vi "twoWire_Resistance_test.vi"() -> ()   [LabVIEW 2026]
uses:
  <vilib>/regexp/Match Regular Expression.xnode
panel:
  out "R (Ohm)":dbl
  in  "VISA resource name":refnum<visa-resource-name>
  out "raw response":string
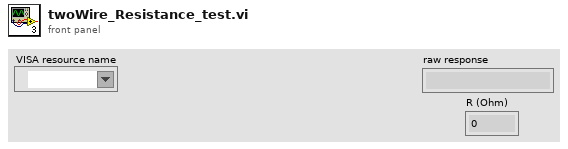
[diagram p1: front panel]
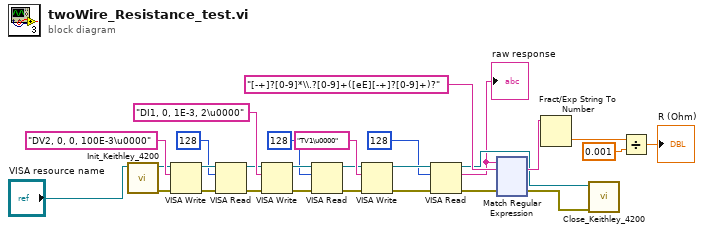
[diagram p0: block diagram]
diagram:
  n1 = call "Init_Keithley_4200.vi"("VISA resource name"="VISA resource name") -> ("error out"=w12:errorcluster, "VISA resource name out"=w13:refnum<visa-resource-name>)  [unwired: 9 in]
  n2 = VISA Write(VISA resource name=w13, write buffer="DV2, 0, 0, 100E-3\u0000", error in (no error)=w12) -> (VISA resource name out=w16:refnum<visa-resource-name>, error out=w15:errorcluster)  [unwired: 1 out]
  n3 = VISA Read(VISA resource name=w16, byte count=u32 128, error in (no error)=w15) -> (VISA resource name out=w11:refnum<visa-resource-name>, error out=w10:errorcluster)  [unwired: 2 out]
  n4 = VISA Write(VISA resource name=w11, write buffer="DI1, 0, 1E-3, 2\u0000", error in (no error)=w10) -> (VISA resource name out=w22:refnum<visa-resource-name>, error out=w21:errorcluster)  [unwired: 1 out]
  n5 = VISA Read(VISA resource name=w22, byte count=u32 128, error in (no error)=w21) -> (VISA resource name out=w20:refnum<visa-resource-name>, error out=w19:errorcluster)  [unwired: 2 out]
  n6 = VISA Write(VISA resource name=w20, write buffer="TV1\u0000", error in (no error)=w19) -> (VISA resource name out=w28:refnum<visa-resource-name>, error out=w27:errorcluster)  [unwired: 1 out]
  n7 = VISA Read(VISA resource name=w28, byte count=u32 128, error in (no error)=w27) -> (VISA resource name out=w7:refnum<visa-resource-name>, read buffer=w1:string, error out=w3:errorcluster)  [unwired: 1 out]
  "raw response" <- w1
  n8 = xnode "Match Regular Expression"("input string"=w1, "regular expression"="[-+]?[0-9]*\\.?[0-9]+([eE][-+]?[0-9]+)?", "error in"=w3) -> ("whole match"=w9:string, "error out"=w2:errorcluster)  [unwired: 3 in, 3 out]
  n9 = Fract/Exp String To Number(string=w9) -> (number=w6:dbl)  [unwired: 3 in, 1 out]
  n10 = call "Close_Keithley_4200.vi"("error in (no error)"=w2, "VISA resource name"=w7) -> ()  [unwired: 9 in, 1 out]
  n11 = Divide(x=w6, y=0.001) -> (x/y=→"R (Ohm)":dbl)
